vi "RC Enum to RC Object.vi"(8 "error in (no error)":errorcluster, 11 "RC Type":T1) -> (0 "error out":errorcluster, 3 "RemoteControl out":refnum<class "RemoteControl.lvclass">)   [LabVIEW 2019, in "RemoteControl.lvclass"]
uses:
  RemoteControl.lvclass
  Typedefs/RC Com Type--enum.ctl
  RemoteControl.ZMQ/RemoteControl.ZMQ.lvclass
  C:/Users/patrick/Documents/GitHub/Instrument-Framework/lvsrc/SMOs/RemoteControl/RemoteControl.lvclass
  RemoteControl.STM/RemoteControl.STM.lvclass
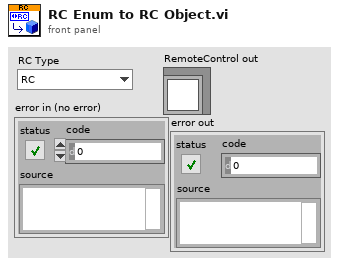
[diagram p1: front panel]
types:
  T1 = typedef "RemoteControl.lvclass/RC Com Type--enum.ctl" = enum16{"RC", "STM", "ZMQ"}
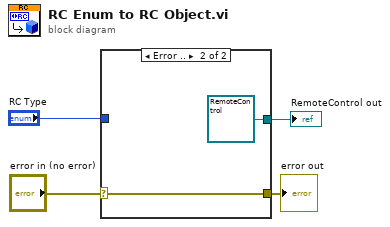
[diagram p0: block diagram]
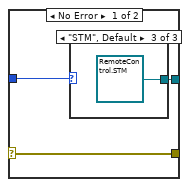
[diagram p2: hidden frame]
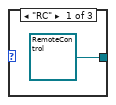
[diagram p3: hidden frame]
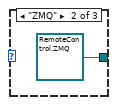
[diagram p4: hidden frame]
diagram:
  n1 = case shown="Error .." "error in (no error)" {
    selector: "error in (no error)" -> [w5 w12]
    tunnel: "RC Type" -> [w7 _]
    tunnel: [w6 refnum<class "RemoteControl.lvclass"> refnum ("RemoteControl in")] -> w3
    tunnel: [w5 w12] -> w1
    frame No Error {
      n2 = case shown="\"STM\", Default" w7 {
        tunnel: [refnum<class "RemoteControl.lvclass"> refnum ("RemoteControl in") refnum<class "RemoteControl.ZMQ.lvclass"> refnum ("RemoteControl.ZMQ.lvclass") refnum<class "RemoteControl.STM.lvclass"> refnum ("RemoteControl.STM.lvclass")] -> w6
        frame "RC" {
        }
        frame "ZMQ" {
        }
        frame "STM", Default {
        }
      }
    }
    frame Error {
    }
  }
  "RemoteControl out" <- w3
  "error out" <- w1
